vi "System_Modeling_LabVIEW_DIP_Elyes_KHECHINE_Ayoub_HEDFI_Elyes_CHAMEKH.vi"() -> ()   [LabVIEW 2022 SP3]
uses:
  <vilib>/imath/engines/lvmath2/RunTimeEngine/IndexRead/NIMS M(S,S).vi
  <instcachedir>/0/NIMS M(S,S)_AC51E74150A542F7991B9634C66F3096.lvgen/NIMS M(S,S)_AC51E74150A542F7991B9634C66F3096_000.vi
  <vilib>/imath/engines/lvmath2/RunTimeEngine/IndexRead/NIMS V(S).vi
  <instcachedir>/0/NIMS V(S)_0488751826AF41519A22953C041130DC.lvgen/NIMS V(S)_0488751826AF41519A22953C041130DC_000.vi
  <vilib>/imath/engines/lvmath2/RunTimeEngine/IndexReplace/NIMS M(S,S)=S.vi
  <instcachedir>/0/NIMS M(S,S)=S_77070144367643E3BE0C1B8B1DC280C8.lvgen/NIMS M(S,S)=S_77070144367643E3BE0C1B8B1DC280C8_000.vi
  <vilib>/imath/engines/lvmath2/RunTimeEngine/ErrorHandling/NIMS_Create Error From Enums.vi
  <vilib>/imathl/engines/lvmath/Functions/Error Handling/Create Error.vi
  <vilib>/imath/engines/lvmath2/RunTimeEngine/IndexReplace/NIMS V(S)=S.vi
  <instcachedir>/0/NIMS V(S)=S_CA4DEDF18C714BDE919160A1D8CBDFAA.lvgen/NIMS V(S)=S_CA4DEDF18C714BDE919160A1D8CBDFAA_000.vi
  <vilib>/imath/engines/lvmath2/RunTimeEngine/NodeEndStatement/NIMS_NodeEndStatement_Output.vi
  <instcachedir>/0/NIMS_NodeEndStatement_Output_53EC0D466D134D7ABD903AC30B43404B.lvgen/NIMS_NodeEndStatement_Output_53EC0D466D134D7ABD903AC30B43404B_002.vi
  <vilib>/imath/engines/lvmath2/RunTimeEngine/ErrorHandling/NIMS_Finalize Error.vi
  <vilib>/addons/Control Design/_Model Construction/Model Creation.llb/Model Creation SubVI/cd_Create State Space Model.vi
  <vilib>/addons/Control Design/_Model Construction/Model File IO.llb/Model File IO Subvi/cd_Write Model to File (SS).vi
  <vilib>/addons/Control Design/_Dynamic Analysis/Dynamic Analysis.llb/Dynamic Analysis subVI/cd_Pole-Zero Map (State-Space).vi
  <vilib>/addons/Control Design/_Utility/Model Viewer.llb/Model Viewer SubVI/cd_Draw State-Space Equation (SS).vi
  <vilib>/addons/Control Design/_Model Construction/NI_LinSys_Model Creation.lvlib
  <vilib>/addons/Control Design/_Utility/NI_CD_Model Viewer.lvlib
  <vilib>/addons/Control Design/_Dynamic Analysis/NI_CD_Dynamic Analysis.lvlib
  <vilib>/addons/Control Design/_Model Construction/NI_LinSys_Model File IO.lvlib
panel:
  in  "Short Pendulum Parameters":T1={"Mp1 (kg)"=0.072, "Lp1 (m)"=0.2095, "Bp1 (N.m.s/rad)"=0.0024, "Jp1 (kg.m^2)"=0.00026347, "lp1 (m)"=0.1143}
  in  "Medium Pendulum Parameters":T2={"Mp2 (kg)"=0.127, "lp2 (m)"=0.1778, "Bp2 (N.m.s/rad)"=0.0024, "Jp2 (kg.m^2)"=0.0012, "Lp2 (m)"=0.3365}
  in  "Motor Parameters":T3={"Rm (Ohm)"=2.6, "Kt (N-m/A)"=0.00767, "Km (V-s/rad)"=0.00767, "Kg"=3.71, "eta_m"=1.0, "eta_g"=1.0, "r_mp (m)"=0.00635}
  in  "IP02 and DBPEN-LIN Parameters":T4={"Mc (kg)"=0.7, "Beq (N-s/m)"=4.3, "Mh (kg)"=0.17}
  in  "Model Name":string="model"
  in  "Save Model":bool
  in  "Stop Button":bool
  out "Poles":cdb[](array[numeric])=[-0.12046012625208034+10.260716470657208i, -0.12046012625208034-10.260716470657208i, -14.286386400967146+0.0i, 6.309365307732558+0.0i, -4.014645359213837+0.0i, 0.0+0.0i, 0.0+0.0i] format="%.4f"
  out "Pole-Zero Map":cluster{dbl[], dbl[]}[](graph)=[{[-0.12046012625208034, -0.12046012625208034, -14.286386400967146, 6.309365307732558, -4.014645359213837, 0.0, 0.0], [10.260716470657208, -10.260716470657208, 0.0, 0.0, 0.0, 0.0, 0.0]}, {[-2.618213552393617e-16], [0.0]}]
  out "State-Space Equation":picture
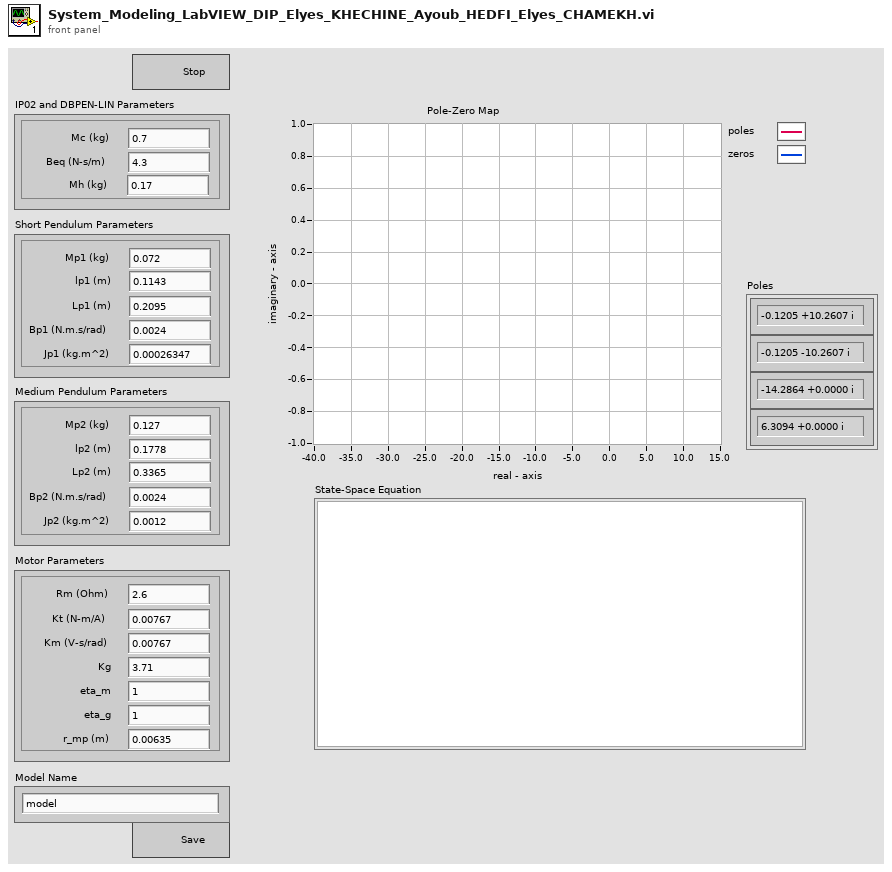
[diagram p1: front panel]
types:
  T1 = cluster{"Mp1 (kg)":dbl, "Lp1 (m)":dbl, "Bp1 (N.m.s/rad)":dbl, "Jp1 (kg.m^2)":dbl, "lp1 (m)":dbl}
  T2 = cluster{"Mp2 (kg)":dbl, "lp2 (m)":dbl, "Bp2 (N.m.s/rad)":dbl, "Jp2 (kg.m^2)":dbl, "Lp2 (m)":dbl}
  T3 = cluster{"Rm (Ohm)":dbl, "Kt (N-m/A)":dbl, "Km (V-s/rad)":dbl, "Kg":dbl, "eta_m":dbl, "eta_g":dbl, "r_mp (m)":dbl}
  T4 = cluster{"Mc (kg)":dbl, "Beq (N-s/m)":dbl, "Mh (kg)":dbl}
  T5 = typedef "NI_LinSys_Model Typedefs.lvlib/CD State Space Model (MIMO).ctl" = cluster{"properties":T6, "A":dbl[][], "B":dbl[][], "C":dbl[][], "D":dbl[][], "StateNames":string[], "Transport Delay":dbl[][]}
  T6 = typedef "NI_LinSys_Model Typedefs.lvlib/CD General Elements.ctl" = cluster{"Model name":string, "Input names":string[], "Output names":string[], "Input Delays":dbl[], "Output Delays":dbl[], "Sampling Time":dbl, "Notes":string}
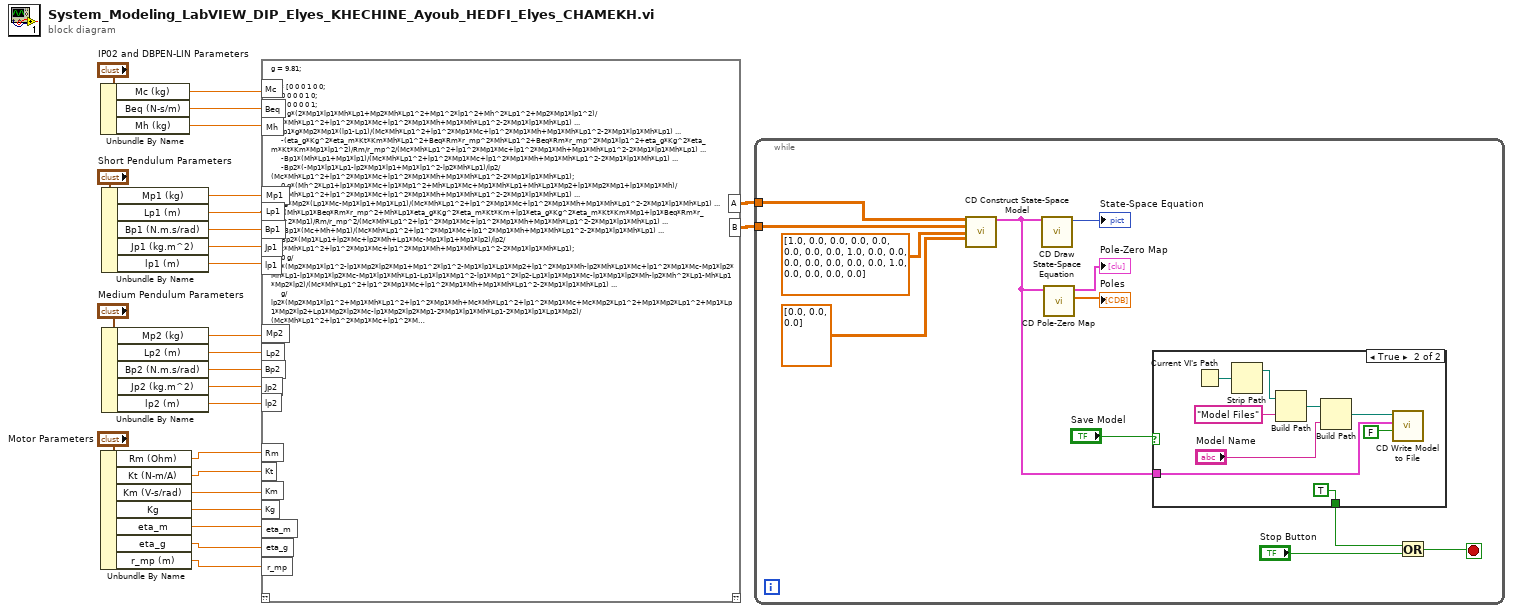
[diagram p0: block diagram]
diagram:
  n1 = Unbundle By Name("IP02 and DBPEN-LIN Parameters") -> ("Mc (kg)"=w24:dbl, "Beq (N-s/m)"=w8:dbl, "Mh (kg)"=w2:dbl)
  n2 = Unbundle By Name("Motor Parameters") -> ("Rm (Ohm)"=w23:dbl, "Kt (N-m/A)"=w22:dbl, "Km (V-s/rad)"=w21:dbl, "Kg"=w20:dbl, "eta_m"=w19:dbl, "eta_g"=w18:dbl, "r_mp (m)"=w17:dbl)
  n3 = Unbundle By Name("Short Pendulum Parameters") -> ("Mp1 (kg)"=w11:dbl, "Lp1 (m)"=w10:dbl, "Bp1 (N.m.s/rad)"=w9:dbl, "Jp1 (kg.m^2)"=w6:dbl, "lp1 (m)"=w5:dbl)
  n4 = Unbundle By Name("Medium Pendulum Parameters") -> ("Mp2 (kg)"=w14:dbl, "Lp2 (m)"=w3:dbl, "Bp2 (N.m.s/rad)"=w13:dbl, "Jp2 (kg.m^2)"=w7:dbl, "lp2 (m)"=w4:dbl)
  n5 = mathscript code="g = 9.81;\n\nA = [0 0 0 1 0 0;\n     0 0 0 0 1 0;\n     0 0 0 0 0 1;\n     0 g*(2*Mp1*lp1*Mh*Lp1+Mp2*Mh*Lp1^2+Mp1^2*lp1^2+Mh^2*Lp1^2+Mp2*Mp1*lp1^2)/(Mc*Mh*Lp1^2+lp1^2*Mp1*Mc+lp1^2*Mp1*Mh+Mp1*Mh*Lp1^2-2*Mp1*lp1*Mh*Lp1) ...\n     lp1*g*Mp2*Mp1*(lp1-Lp1)/(Mc*Mh*Lp1^2+lp1^2*Mp1*Mc+lp1^2*Mp1*Mh+Mp1*Mh*Lp1^2-2*Mp1*lp1*Mh*Lp1) ...\n     -(eta_g*Kg^2*eta_m*Kt*Km*Mh*Lp1^2+Beq*Rm*r_mp^2*Mh*Lp1^2+Beq*Rm*r_mp^2*Mp1*lp1^2+eta_g*Kg^2*eta_m*Kt*Km*Mp1*lp1^2)/Rm/r_mp^2/(Mc*Mh*Lp1^2+lp1^2*Mp1*Mc+lp1^2*Mp1*Mh+Mp1*Mh*Lp1^2-2*Mp1*lp1*Mh*Lp1) ...\n     -Bp1*(Mh*Lp1+Mp1*lp1)/(Mc*Mh*Lp1^2+lp1^2*Mp1*Mc+lp1^2*Mp1*Mh+Mp1*Mh*Lp1^2-2*Mp1*lp1*Mh*Lp1) ...\n     -Bp2*(-Mp1*lp1*Lp1-lp2*Mp1*lp1+Mp1*lp1^2-lp2*Mh*Lp1)/lp2/(Mc*Mh*Lp1^2+lp1^2*Mp1*Mc+lp1^2*Mp1*Mh+Mp1*Mh*Lp1^2-2*Mp1*lp1*Mh*Lp1);\n     0 g*(Mh^2*Lp1+lp1*Mp1*Mc+lp1*Mp1^2+Mh*Lp1*Mc+Mp1*Mh*Lp1+Mh*Lp1*Mp2+lp1*Mp2*Mp1+lp1*Mp1*Mh)/(Mc*Mh*Lp1^2+lp1^2*Mp1*Mc+lp1^2*Mp1*Mh+Mp1*Mh*Lp1^2-2*Mp1*lp1*Mh*Lp1) ...\n     -g*Mp2*(Lp1*Mc-Mp1*lp1+Mp1*Lp1)/(Mc*Mh*Lp1^2+lp1^2*Mp1*Mc+lp1^2*Mp1*Mh+Mp1*Mh*Lp1^2-2*Mp1*lp1*Mh*Lp1) ...\n     -(Mh*Lp1*Beq*Rm*r_mp^2+Mh*Lp1*eta_g*Kg^2*eta_m*Kt*Km+lp1*eta_g*Kg^2*eta_m*Kt*Km*Mp1+lp1*Beq*Rm*r_mp^2*Mp1)/Rm/r_mp^2/(Mc*Mh*Lp1^2+lp1^2*Mp1*Mc+lp1^2*Mp1*Mh+Mp1*Mh*Lp1^2-2*Mp1*lp1*Mh*Lp1) ...\n     -Bp1*(Mc+Mh+Mp1)/(Mc*Mh*Lp1^2+lp1^2*Mp1*Mc+lp1^2*Mp1*Mh+Mp1*Mh*Lp1^2-2*Mp1*lp1*Mh*Lp1) ...\n     Bp2*(Mp1*Lp1+lp2*Mc+lp2*Mh+Lp1*Mc-Mp1*lp1+Mp1*lp2)/lp2/(Mc*Mh*Lp1^2+lp1^2*Mp1*Mc+lp1^2*Mp1*Mh+Mp1*Mh*Lp1^2-2*Mp1*lp1*Mh*Lp1);\n     0 g/lp2*(Mp2*Mp1*lp1^2-lp1*Mp2*lp2*Mp1+Mp1^2*lp1^2-Mp1*lp1*Lp1*Mp2+lp1^2*Mp1*Mh-lp2*Mh*Lp1*Mc+lp1^2*Mp1*Mc-Mp1*lp2*Mh*Lp1-lp1*Mp1*lp2*Mc-Mp1*lp1*Mh*Lp1-Lp1*lp1*Mp1^2-lp1*Mp1^2*lp2-Lp1*lp1*Mp1*Mc-lp1*Mp1*lp2*Mh-lp2*Mh^2*Lp1-Mh*Lp1*Mp2*lp2)/(Mc*Mh*Lp1^2+lp1^2*Mp1*Mc+lp1^2*Mp1*Mh+Mp1*Mh*Lp1^2-2*Mp1*lp1*Mh*Lp1) ...\n     g/lp2*(Mp2*Mp1*lp1^2+Mp1*Mh*Lp1^2+lp1^2*Mp1*Mh+Mc*Mh*Lp1^2+lp1^2*Mp1*Mc+Mc*Mp2*Lp1^2+Mp1*Mp2*Lp1^2+Mp1*Lp1*Mp2*lp2+Lp1*Mp2*lp2*Mc-lp1*Mp2*lp2*Mp1-2*Mp1*lp1*Mh*Lp1-2*Mp1*lp1*Lp1*Mp2)/(Mc*Mh*Lp1^2+lp1^2*Mp1*Mc+lp1^2*Mp1*Mh+Mp1*Mh*Lp1^2-2*Mp1*lp1*Mh*Lp1) ...\n     -1/lp2*(-lp1*eta_g*Kg^2*eta_m*Kt*Km*lp2*Mp1+eta_g*Kg^2*eta_m*Kt*Km*Mp1*lp1^2-lp1*Beq*Rm*r_mp^2*lp2*Mp1-Lp1*lp1*Beq*Rm*r_mp^2*Mp1-Lp1*lp1*eta_g*Kg^2*eta_m*Kt*Km*Mp1-Mh*Lp1*eta_g*Kg^2*eta_m*Kt*Km*lp2-Mh*Lp1*Beq*Rm*r_mp^2*lp2+Beq*Rm*r_mp^2*Mp1*lp1^2)/Rm/r_mp^2/(Mc*Mh*Lp1^2+lp1^2*Mp1*Mc+lp1^2*Mp1*Mh+Mp1*Mh*Lp1^2-2*Mp1*lp1*Mh*Lp1) ...\n     1/lp2*Bp1*(Mp1*Lp1+lp2*Mc+lp2*Mh+Lp1*Mc-Mp1*lp1+Mp1*lp2)/(Mc*Mh*Lp1^2+lp1^2*Mp1*Mc+lp1^2*Mp1*Mh+Mp1*Mh*Lp1^2-2*Mp1*lp1*Mh*Lp1) ...\n     -Bp2*(lp1^2*Mp1*Mc+lp2^2*Mp2*Mh+lp2^2*Mp2*Mp1+lp2^2*Mp2*Mc+lp1^2*Mp1*Mh-2*lp1*Mp2*lp2*Mp1-2*Mp1*lp1*Mh*Lp1+Mp2*Mp1*lp1^2+2*Mp1*Lp1*Mp2*lp2+2*Lp1*Mp2*lp2*Mc+Mc*Mh*Lp1^2+Mc*Mp2*Lp1^2+Mp1*Mh*Lp1^2+Mp1*Mp2*Lp1^2-2*Mp1*lp1*Lp1*Mp2)/lp2^2/Mp2/(Mc*Mh*Lp1^2+lp1^2*Mp1*Mc+lp1^2*Mp1*Mh+Mp1*Mh*Lp1^2-2*Mp1*lp1*Mh*Lp1)];\n     \n     B = [0; 0; 0; eta_g*Kg*eta_m*Kt/r_mp*(Mh*Lp1^2+Mp1*lp1^2)/Rm/(Mc*Mh*Lp1^2+lp1^2*Mp1*Mc+lp1^2*Mp1*Mh+Mp1*Mh*Lp1^2-2*Mp1*lp1*Mh*Lp1);...\n         eta_g*Kg*eta_m*Kt/r_mp*(Mh*Lp1+Mp1*lp1)/Rm/(Mc*Mh*Lp1^2+lp1^2*Mp1*Mc+lp1^2*Mp1*Mh+Mp1*Mh*Lp1^2-2*Mp1*lp1*Mh*Lp1);...\n         eta_g*Kg*eta_m*Kt/r_mp/lp2*(-Mp1*lp1*Lp1-lp2*Mp1*lp1+Mp1*lp1^2-lp2*Mh*Lp1)/Rm/(Mc*Mh*Lp1^2+lp1^2*Mp1*Mc+lp1^2*Mp1*Mh+Mp1*Mh*Lp1^2-2*Mp1*lp1*Mh*Lp1)];\n     C = eye(3,6);\n     D = zeros(3,1);\n\n%Actuator Dynamics\nA(4,4) = A(4,4) - B(4)*eta_g*Kg^2*eta_m*Kt*Km/r_mp^2/Rm;\nA(5,4) = A(5,4) - B(5)*eta_g*Kg^2*eta_m*Kt*Km/r_mp^2/Rm;\nA(6,4) = A(6,4) - B(6)*eta_g*Kg^2*eta_m*Kt*Km/r_mp^2/Rm;\nB = eta_g*Kg*eta_m*Kt/r_mp/Rm*B;\n\n%Add Integrator State\n    A(7,1) = 1;\n    A(7,7) = 0;\n    B(7) = 0;\n    C = eye(3,7);"("Mc"=w24, "Beq"=w8, "Kg"=w20, "Km"=w21, "Kt"=w22, "Rm"=w23, "eta_m"=w19, "eta_g"=w18, "r_mp"=w17, "Mp2"=w14, "Lp2"=w3, "Bp2"=w13, "Mp1"=w11, "Lp1"=w10, "Bp1"=w9, "Jp1"=w6, "Jp2"=w7, "lp1"=w5, "lp2"=w4, "Mh"=w2) -> ("A"=w16:dbl[][], "B"=w15:dbl[][])  [unwired: 1 in, 1 out]
  n6 = while {
    tunnel: w16 -> [w28]
    tunnel: w15 -> [w27]
    stop <- w31 stop-if-true
    n7 = call-poly <vilib>:"CD Construct State-Space Model.vi"("A"=w28, "B"=w27, "C"=dbl[][] [[1.0, 0.0, 0.0, 0.0, 0.0, 0.0, 0.0], [0.0, 1.0, 0.0, 0.0, 0.0, 0.0, 0.0], [0.0, 0.0, 1.0, 0.0, 0.0, 0.0, 0.0]], "D"=dbl[][] [[0.0], [0.0], [0.0]]) -> ("State-Space Model"=w32:T5)  [unwired: 10 in, 1 out]
    n8 = call-poly <vilib>:"CD Draw State-Space Equation.vi"("State-Space Model"=w32) -> ("Equation"=→"State-Space Equation":picture)  [unwired: 8 in, 2 out]
    n9 = call-poly <vilib>:"CD Pole-Zero Map.vi"("State-Space Model"=w32) -> ("Poles"=→"Poles":cdb[], "Pole-Zero Map"=→"Pole-Zero Map":cluster{dbl[], dbl[]}[])  [unwired: 7 in, 2 out]
    n10 = case shown="True" "Save Model" {
      tunnel: w32 -> [_ w41]
      tunnel: [_ TRUE] -> w30
      frame False {
      }
      frame True {
        n11 = Current VI's Path() -> (path=w42:path)
        n12 = Strip Path(path=w42) -> (stripped path=w45:path)  [unwired: 1 out]
        n13 = Build Path(base path=w45, name or relative path="Model Files") -> (appended path=w46:path)
        n14 = Build Path(base path=w46, name or relative path="Model Name") -> (appended path=w43:path)
        n15 = call-poly <vilib>:"CD Write Model to File.vi"("Append to File? (new file:F)"=FALSE, "State-Space Model"=w41, "File Path (dialog if empty)"=w43) -> ()  [unwired: 6 in, 3 out]
      }
    }
    n16 = Or(x=w30, y="Stop Button") -> (x .or. y?=w31:bool)
  }
